vi "Multi Dut Cmd Setting.vi"(8 "error in (no error)":errorcluster, 9 "Test Seq":i32(ring) items=["C1_C2_C3", "C2_C1_C3", "C3_C2_C1"], 10 "Cmin/Act":bool=TRUE, 11 "WS1050/51":bool=TRUE) -> (0 "error out":errorcluster, 1 "Cmd 3":string[](array[string]), 2 "Name 3":string[](array[string]), 3 "Name Header":string[](array[string]), 4 "Cmd 2":string[](array[string]), 5 "Name 2":string[](array[string]), 6 "Cmd 1":string[](array[string]), 7 "Name 1":string[](array[string]))   [LabVIEW 2012]
panel:
  in  "Cmd 51 Cmin":string[](array[string])=["00", "00", "00", "00", "00", "00", "00", "00", "00", "00", "00", "00", "00", "00", "00", "00", "00", "00", "00", "00", "00", "00", "00", "00", "00", "00", "00", "00", "00"]
  in  "Cmd 50 Cmin":string[](array[string])=["00", "00", "00", "00", "00", "00", "00", "00", "00", "00", "00", "00", "00", "00", "00", "00", "00", "00", "00", "00", "00", "00", "00", "00", "00", "00", "00", "00", "00", "00", "00", "00", "00", "00", "00"]
  in  "Cmd 51":string[](array[string])=["00", "01", "00", "02", "00", "04", "00", "08", "04", "0C", "08", "10", "0C", "14", "10", "18", "14", "1C", "18", "20", "1C", "24", "20", "28", "24", "2C", "28", "2F", "00"]
  in  "Name 51":string[](array[string])=["Min", "F1", "F1_OFF", "F2", "F2_OFF", "S1", "S1_OFF", "S2", "S2_OFF", "S3", "S3_OFF", "S4", "S4_OFF", "S5", "S5_OFF", "S6", "S6_OFF", "S7", "S7_OFF", "S8", "S8_OFF", "S9", "S9_OFF", "S10", "S10_OFF", "S11", "S11_OFF", "S11_F12", "Min2"]
  in  "Cmd 50":string[](array[string])=["00", "01", "00", "02", "00", "04", "00", "08", "04", "0C", "08", "10", "0C", "14", "10", "18", "14", "1C", "18", "20", "1C", "24", "20", "28", "24", "2C", "28", "30", "2C", "34", "30", "38", "34", "3B", "00"]
  in  "Name 50":string[](array[string])=["Min", "F1", "F1_OFF", "F2", "F2_OFF", "S1", "S1_OFF", "S2", "S2_OFF", "S3", "S3_OFF", "S4", "S4_OFF", "S5", "S5_OFF", "S6", "S6_OFF", "S7", "S7_OFF", "S8", "S8_OFF", "S9", "S9_OFF", "S10", "S10_OFF", "S11", "S11_OFF", "S12", "S12_OFF", "S13", "S13_OFF", "S14", "S14_OFF", "S14F12", "Min2"]
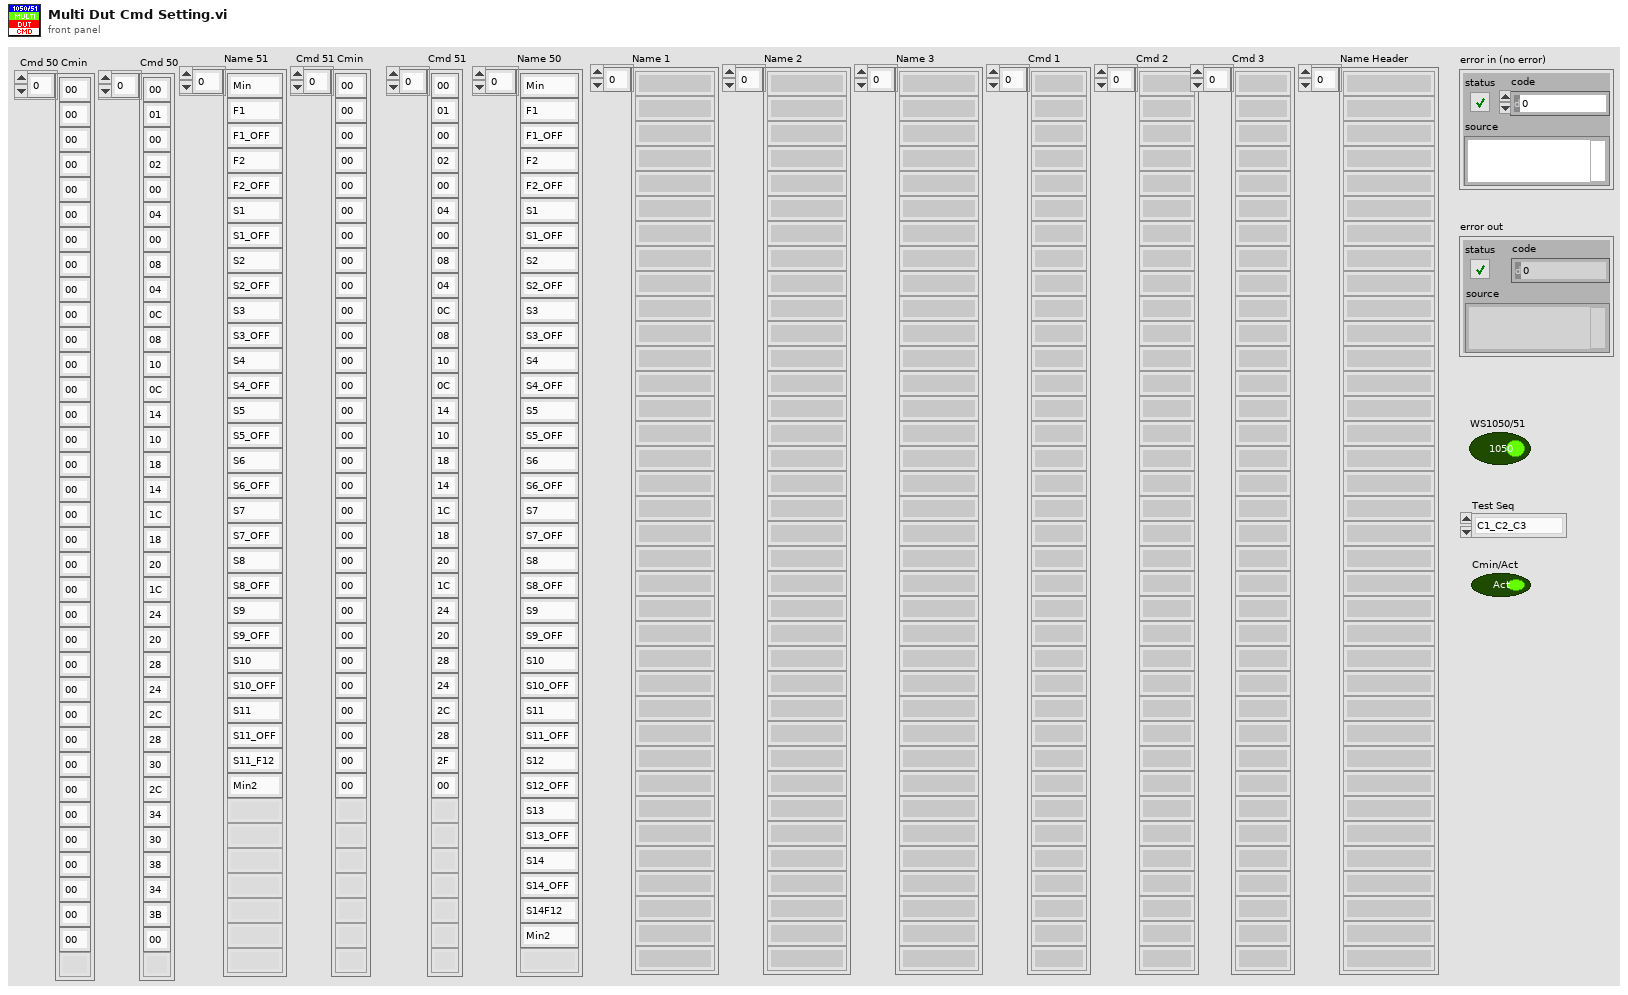
[diagram p1: front panel]
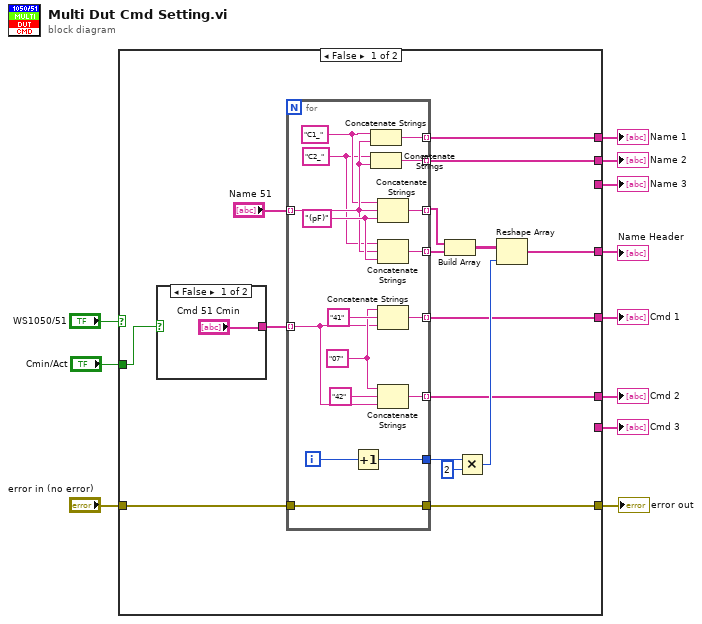
[diagram p0: block diagram]
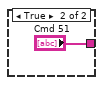
[diagram p2: hidden frame]
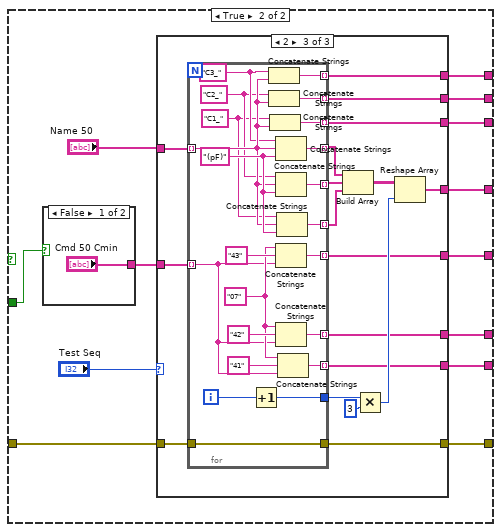
[diagram p3: hidden frame]
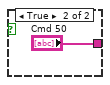
[diagram p4: hidden frame]
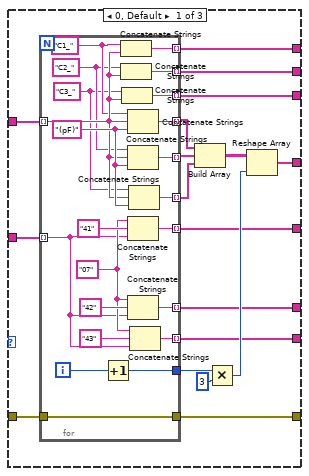
[diagram p5: hidden frame]
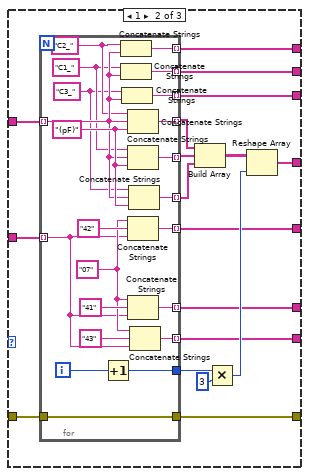
[diagram p6: hidden frame]
diagram:
  n1 = case shown="False" "WS1050/51" {
    tunnel: "error in (no error)" -> [w16 w59]
    tunnel: [w15 w58] -> w10
    tunnel: [w19 w57] -> w8
    tunnel: [w21 w56] -> w7
    tunnel: [w20 w55] -> w6
    tunnel: [_ w54] -> w5
    tunnel: [w14 w53] -> w4
    tunnel: [w13 w52] -> w3
    tunnel: [_ w51] -> w2
    tunnel: "Cmin/Act" -> [w12 w47]
    frame False {
      n2 = case shown="False" w12 {
        tunnel: ["Cmd 51 Cmin" "Cmd 51"] -> w17
        frame False {
        }
        frame True {
        }
      }
      n3 = for {
        tunnel: "Name 51" -> [w33] mode=indexing
        tunnel: [w46] -> w22 mode=indexing
        tunnel: [w45] -> w23 mode=indexing
        tunnel: w17 -> [w39] mode=indexing
        tunnel: [w43] -> w14 mode=indexing
        tunnel: [w41] -> w13 mode=indexing
        tunnel: [w35] -> w21 mode=indexing
        tunnel: [w37] -> w26
        tunnel: [w34] -> w20 mode=indexing
        tunnel: w16 -> [w30]
        tunnel: [w30] -> w15
        i -> [w36]
        w31 = "C2_" ("string")
        w38 = "(pF)" ("string")
        w32 = "C1_" ("string")
        w40 = "07" ("string")
        n4 = Increment(x=w36) -> (x+1=w37:i32)
        n5 = Concatenate Strings(w32, w33) -> (w35:string)
        n6 = Concatenate Strings(w31, w33) -> (w34:string)
        n7 = Concatenate Strings(w32, w33, w38) -> (w46:string)
        n8 = Concatenate Strings(w31, w33, w38) -> (w45:string)
        n9 = Concatenate Strings(w40, "41" ("string"), w39) -> (w43:string)
        n10 = Concatenate Strings(w40, "42" ("string"), w39) -> (w41:string)
      }
      n11 = Build Array(w22, w23) -> (w24:string[][])
      n12 = Multiply(x=w26, y=2) -> (x*y=w25:i32)
      n13 = Reshape Array(w24, w25) -> (w19:string[])
    }
    frame True {
      n14 = case shown="False" w47 {
        tunnel: ["Cmd 50 Cmin" "Cmd 50"] -> w48
        frame False {
        }
        frame True {
        }
      }
      n15 = case shown="2" "Test Seq" {
        tunnel: "Name 50" -> [w79 w119 w159]
        tunnel: w48 -> [w78 w118 w158]
        tunnel: w59 -> [w70 w110 w150]
        tunnel: [w69 w109 w149] -> w58
        tunnel: [w68 w108 w148] -> w57
        tunnel: [w67 w107 w147] -> w56
        tunnel: [w66 w106 w146] -> w55
        tunnel: [w65 w105 w145] -> w54
        tunnel: [w64 w104 w144] -> w53
        tunnel: [w63 w103 w143] -> w52
        tunnel: [w62 w102 w142] -> w51
        frame 0, Default {
          n16 = for {
            tunnel: w79 -> [w85] mode=indexing
            tunnel: [w101] -> w77 mode=indexing
            tunnel: [w100] -> w76 mode=indexing
            tunnel: [w99] -> w75 mode=indexing
            tunnel: w78 -> [w92] mode=indexing
            tunnel: [w97] -> w64 mode=indexing
            tunnel: [w95] -> w63 mode=indexing
            tunnel: [w91] -> w62 mode=indexing
            tunnel: [w87] -> w67 mode=indexing
            tunnel: [w89] -> w72
            tunnel: [w86] -> w66 mode=indexing
            tunnel: [w84] -> w65 mode=indexing
            tunnel: w70 -> [w80]
            tunnel: [w80] -> w69
            i -> [w88]
            w81 = "C3_" ("string")
            w82 = "C2_" ("string")
            w90 = "(pF)" ("string")
            w83 = "C1_" ("string")
            w94 = "07" ("string")
            n17 = Increment(x=w88) -> (x+1=w89:i32)
            n18 = Concatenate Strings(w83, w85) -> (w87:string)
            n19 = Concatenate Strings(w82, w85) -> (w86:string)
            n20 = Concatenate Strings(w81, w85) -> (w84:string)
            n21 = Concatenate Strings(w83, w85, w90) -> (w101:string)
            n22 = Concatenate Strings(w82, w85, w90) -> (w100:string)
            n23 = Concatenate Strings(w94, "41" ("string"), w92) -> (w97:string)
            n24 = Concatenate Strings(w94, "42" ("string"), w92) -> (w95:string)
            n25 = Concatenate Strings(w81, w85, w90) -> (w99:string)
            n26 = Concatenate Strings(w94, "43" ("string"), w92) -> (w91:string)
          }
          n27 = Build Array(w77, w76, w75) -> (w74:string[][])
          n28 = Multiply(x=w72, y=3) -> (x*y=w73:i32)
          n29 = Reshape Array(w74, w73) -> (w68:string[])
        }
        frame 1 {
          n30 = for {
            tunnel: w119 -> [w125] mode=indexing
            tunnel: [w141] -> w117 mode=indexing
            tunnel: [w140] -> w116 mode=indexing
            tunnel: [w139] -> w115 mode=indexing
            tunnel: w118 -> [w132] mode=indexing
            tunnel: [w137] -> w104 mode=indexing
            tunnel: [w135] -> w103 mode=indexing
            tunnel: [w131] -> w102 mode=indexing
            tunnel: [w127] -> w107 mode=indexing
            tunnel: [w129] -> w112
            tunnel: [w126] -> w106 mode=indexing
            tunnel: [w124] -> w105 mode=indexing
            tunnel: w110 -> [w120]
            tunnel: [w120] -> w109
            i -> [w128]
            w121 = "C3_" ("string")
            w122 = "C1_" ("string")
            w130 = "(pF)" ("string")
            w123 = "C2_" ("string")
            w134 = "07" ("string")
            n31 = Increment(x=w128) -> (x+1=w129:i32)
            n32 = Concatenate Strings(w123, w125) -> (w127:string)
            n33 = Concatenate Strings(w122, w125) -> (w126:string)
            n34 = Concatenate Strings(w121, w125) -> (w124:string)
            n35 = Concatenate Strings(w123, w125, w130) -> (w141:string)
            n36 = Concatenate Strings(w122, w125, w130) -> (w140:string)
            n37 = Concatenate Strings(w134, "42" ("string"), w132) -> (w137:string)
            n38 = Concatenate Strings(w134, "41" ("string"), w132) -> (w135:string)
            n39 = Concatenate Strings(w121, w125, w130) -> (w139:string)
            n40 = Concatenate Strings(w134, "43" ("string"), w132) -> (w131:string)
          }
          n41 = Build Array(w117, w116, w115) -> (w114:string[][])
          n42 = Multiply(x=w112, y=3) -> (x*y=w113:i32)
          n43 = Reshape Array(w114, w113) -> (w108:string[])
        }
        frame 2 {
          n44 = for {
            tunnel: w159 -> [w165] mode=indexing
            tunnel: [w181] -> w157 mode=indexing
            tunnel: [w180] -> w156 mode=indexing
            tunnel: [w179] -> w155 mode=indexing
            tunnel: w158 -> [w172] mode=indexing
            tunnel: [w177] -> w144 mode=indexing
            tunnel: [w175] -> w143 mode=indexing
            tunnel: [w171] -> w142 mode=indexing
            tunnel: [w167] -> w147 mode=indexing
            tunnel: [w169] -> w152
            tunnel: [w166] -> w146 mode=indexing
            tunnel: [w164] -> w145 mode=indexing
            tunnel: w150 -> [w160]
            tunnel: [w160] -> w149
            i -> [w168]
            w161 = "C1_" ("string")
            w162 = "C2_" ("string")
            w170 = "(pF)" ("string")
            w163 = "C3_" ("string")
            w174 = "07" ("string")
            n45 = Increment(x=w168) -> (x+1=w169:i32)
            n46 = Concatenate Strings(w163, w165) -> (w167:string)
            n47 = Concatenate Strings(w162, w165) -> (w166:string)
            n48 = Concatenate Strings(w161, w165) -> (w164:string)
            n49 = Concatenate Strings(w163, w165, w170) -> (w181:string)
            n50 = Concatenate Strings(w162, w165, w170) -> (w180:string)
            n51 = Concatenate Strings(w174, "43" ("string"), w172) -> (w177:string)
            n52 = Concatenate Strings(w174, "42" ("string"), w172) -> (w175:string)
            n53 = Concatenate Strings(w161, w165, w170) -> (w179:string)
            n54 = Concatenate Strings(w174, "41" ("string"), w172) -> (w171:string)
          }
          n55 = Build Array(w157, w156, w155) -> (w154:string[][])
          n56 = Multiply(x=w152, y=3) -> (x*y=w153:i32)
          n57 = Reshape Array(w154, w153) -> (w148:string[])
        }
      }
    }
  }
  "error out" <- w10
  "Name Header" <- w8
  "Name 1" <- w7
  "Name 2" <- w6
  "Name 3" <- w5
  "Cmd 1" <- w4
  "Cmd 2" <- w3
  "Cmd 3" <- w2
